vi "Modbus FGV.vi"(8 "error in":errorcluster, 9 "Modbus Set":refnum<class "Modbus.lvclass">, 11 "Action":T1) -> (0 "error out":errorcluster, 3 "Modbus Ref":refnum<class "Modbus.lvclass">)   [LabVIEW 2023, in "HardwareAbstractionLayer_LVOOP.lvlib" / "Modbus.lvclass"]
uses:
  Modbus.lvclass
  Teststand Steptypes/Control/Modubs FGV State.ctl
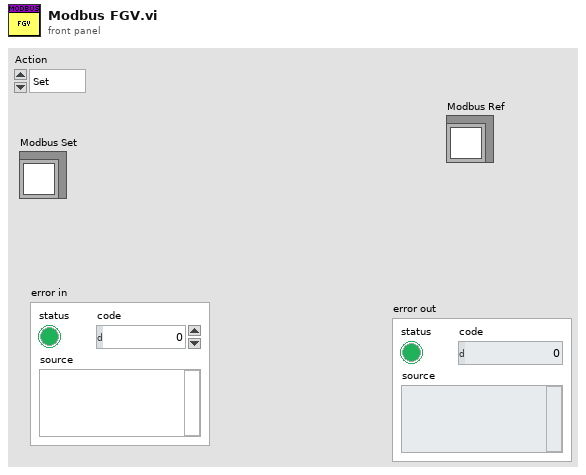
[diagram p1: front panel]
types:
  T1 = typedef "HardwareAbstractionLayer_LVOOP.lvlib/Modbus.lvclass/Modubs FGV State.ctl" = enum16{"Set", "Get"}
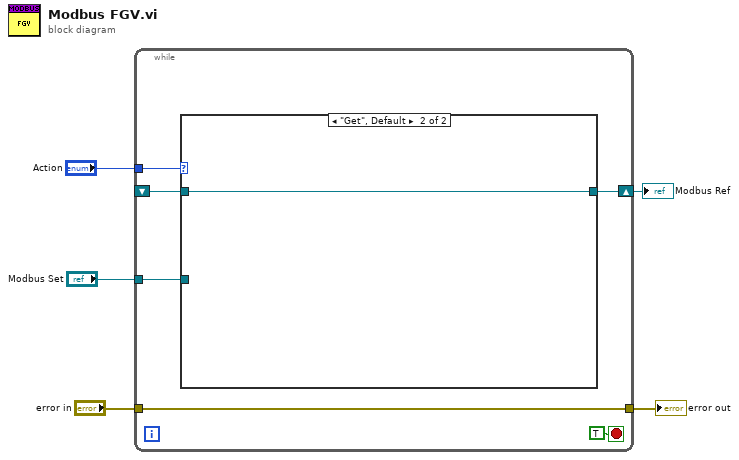
[diagram p0: block diagram]
diagram:
  n1 = while {
    tunnel: "Modbus Set" -> [w10]
    tunnel: "error in" -> [w9]
    tunnel: [w9] -> w3
    tunnel: "Action" -> [w8]
    shift-right: [w7] -> w1
    shift-left: _ -> [w6]
    stop <- TRUE ("stop") stop-if-true
    n2 = case shown="\"Get\", Default" w8 {
      tunnel: w10 -> [w12 _]
      tunnel: [w12 w13] -> w7
      tunnel: w6 -> [_ w13]
      frame "Set" {
      }
      frame "Get", Default {
      }
    }
  }
  "error out" <- w3
  "Modbus Ref" <- w1
